vi "Copy Template Method.vi"(7 "App Inst":refnum<vi>, 8 "error in (no error)":errorcluster, 9 "Method":string, 10 "Template Class":path, 11 "Message Class":refnum<vi>) -> (0 "error out":errorcluster, 1 "Method Reference":refnum<vi>)   [LabVIEW 2020, in "Message Rescripter.lvlib"]
uses:
  Message Rescripter.lvlib
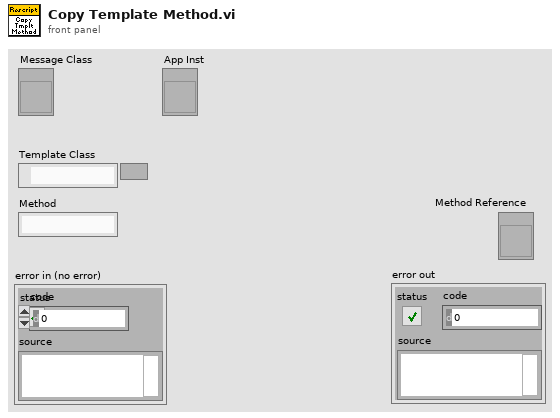
[diagram p1: front panel]
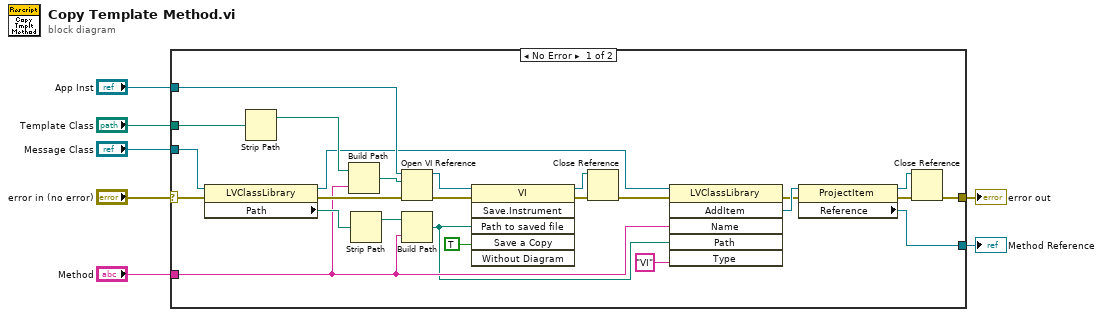
[diagram p0: block diagram]
diagram:
  n1 = case shown="No Error" "error in (no error)" {
    selector: "error in (no error)" -> [w8 w33]
    tunnel: "Message Class" -> [w32 _]
    tunnel: "Template Class" -> [w24 _]
    tunnel: "App Inst" -> [w23 _]
    tunnel: "Method" -> [w17 _]
    tunnel: [w14 w33] -> w3
    tunnel: [w9 _] -> w2
    frame No Error {
      n2 = property class="LVClassLibrary"(reference=w32, error in=w8) -> (reference out=w18:refnum<vi>, error out=w27:errorcluster, "Path"=w31:path)
      n3 = Strip Path(path=w24) -> (stripped path=w19:path)  [unwired: 1 out]
      n4 = Build Path(base path=w19, name or relative path=w17) -> (appended path=w25:path)
      n5 = Strip Path(path=w31) -> (stripped path=w30:path)  [unwired: 1 out]
      n6 = Open VI Reference(application reference (local)=w23, vi path=w25, error in (no error)=w27) -> (vi reference=w20:refnum<vi>, error out=w21:errorcluster)  [unwired: 3 in]
      n7 = Build Path(base path=w30, name or relative path=w17) -> (appended path=w15:path)
      n8 = invoke class="VI" method="Save.Instrument"(reference=w20, error in=w21, "Path to saved file"=w15, "Save a Copy"=TRUE) -> (reference out=w28:refnum<vi>, error out=w29:errorcluster)  [unwired: 2 in, 4 out]
      n9 = Close Reference(reference=w28, error in (no error)=w29) -> (error out=w22:errorcluster)
      n10 = invoke class="LVClassLibrary" method="AddItem"(reference=w18, error in=w22, "Name"=w17, "Path"=w15, "Type"="VI") -> (error out=w12:errorcluster, "AddItem"=w13:refnum<vi>)  [unwired: 1 in, 4 out]
      n11 = property class="ProjectItem"(reference=w13, error in=w12) -> (reference out=w11:refnum<vi>, error out=w10:errorcluster, "Reference"=w9:refnum<vi>)
      n12 = Close Reference(reference=w11, error in (no error)=w10) -> (error out=w14:errorcluster)
    }
    frame Error {
    }
  }
  "error out" <- w3
  "Method Reference" <- w2
